vi "exec.vi"(8 "error in (no error)":errorcluster, 11 "ChangeWavelength in":refnum<class "ChangeWavelength.lvclass">) -> (0 "error out":errorcluster, 3 "ChangeWavelength out":refnum<class "ChangeWavelength.lvclass">)   [LabVIEW 2016, in "ChangeWavelength.lvclass"]
uses:
  ChangeWavelength.lvclass
  C:/Users/aanania/Documents/ts_monochromator_windows/WindowsController/Commands/Command/Command.lvclass
  Command/Command.lvclass/Command.ctl
  ChangeWavelength.lvclass/ChangeWavelength.ctl
  Command/Command.lvclass
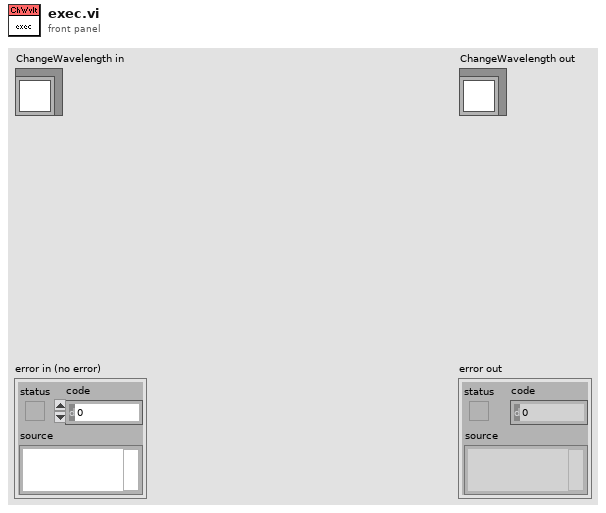
[diagram p1: front panel]
types:
  T1 = typedef "wavelength.ctl" = dbl
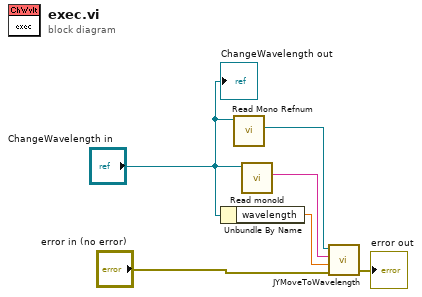
[diagram p0: block diagram]
diagram:
  n1 = Unbundle By Name("ChangeWavelength in") -> ("wavelength"=w4:T1)
  n2 = call "Read Mono Refnum.vi"("Command in"="ChangeWavelength in") -> ("Mono Refnum"=w6:refnum<k7>)  [unwired: 8 in, 2 out]
  n3 = call "Read monoId.vi"("Command in"="ChangeWavelength in") -> ("monoId"=w5:string)  [unwired: 8 in, 2 out]
  n4 = call "JYMoveToWavelength.vi"("error in (no error)"="error in (no error)", "Target WL"=w4, "UniqueID"=w5, "RefNum In"=w6) -> ("error out"=→"error out":errorcluster)  [unwired: 2 out]
  "ChangeWavelength out" <- "ChangeWavelength in"
